vi "Structure Name to Key.vi"(5 "Name":string) -> (2 "Key":string)   [LabVIEW 2019]
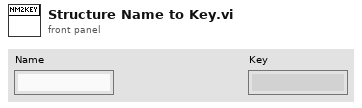
[diagram p1: front panel]
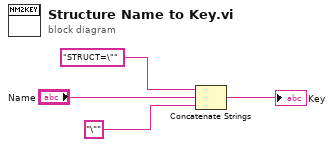
[diagram p0: block diagram]
diagram:
  n1 = Concatenate Strings("STRUCT=\"" ("string"), "Name", "\"" ("string")) -> (→"Key":string)
